vi "Fit.vi"(1 "Array Time":i32[](array[numeric]), 2 "Array BAT Current":dbl[](array[numeric]), 3 "BAT Current":dbl) -> (0 "Coefficients":dbl[](array[numeric]))   [LabVIEW 2015]
uses:
  <vilib>/Analysis/6fits.llb/Curve Fitting Criteria.ctl
  <vilib>/Analysis/NI_AALPro.lvlib
panel:
  in  "method":T1 items=["Least Square", "Least Absolute Residual", "Bisquare"]
  out "Time":i32[](array[numeric])
  out "Current (A)":dbl[](array[numeric])
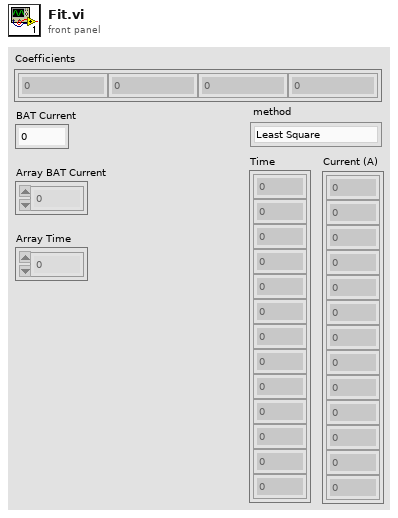
[diagram p1: front panel]
types:
  T1 = typedef "NI_AALPro.lvlib/Curve Fitting Criteria.ctl" = u16
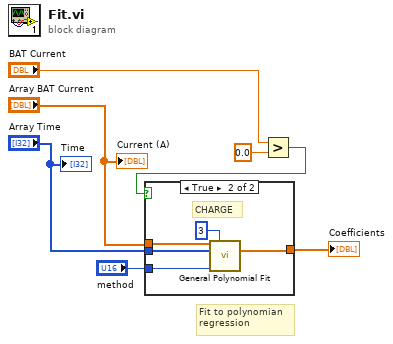
[diagram p0: block diagram]
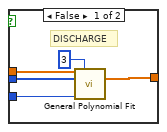
[diagram p2: hidden frame]
diagram:
  # "Fit to polynomian\nregression"
  n1 = Greater?(x="BAT Current", y=0.0) -> (0:w5:bool)
  n2 = case shown="True" w5 {
    tunnel: "Array Time" -> [w11 w16]
    tunnel: "method" -> [w10 w15]
    tunnel: [w9 w13] -> w4
    tunnel: "Array BAT Current" -> [w8 w14]
    frame False {
      # "DISCHARGE"
      n3 = call <vilib>:"General Polynomial Fit.vi"("Y"=w8, "polynomial order"=3, "X"=w11, "method"=w10) -> ("Polynomial Coefficients"=w9:dbl[])  [unwired: 8 in, 3 out]
    }
    frame True {
      # "CHARGE"
      n4 = call <vilib>:"General Polynomial Fit.vi"("Y"=w14, "polynomial order"=3, "X"=w16, "method"=w15) -> ("Polynomial Coefficients"=w13:dbl[])  [unwired: 8 in, 3 out]
    }
  }
  "Coefficients" <- w4
  "Current (A)" <- "Array BAT Current"
  "Time" <- "Array Time"
